vi "Create Image Name.vi"(8 "error in (no error)":errorcluster, 11 "Save Image in":refnum<class "Save Image.lvclass">) -> (0 "error out":errorcluster, 3 "Save Image out":refnum<class "Save Image.lvclass">)   [LabVIEW 2018, in "Save Image.lvclass"]
uses:
  Save Image.lvclass
  Save Image.lvclass/Save Image.ctl
  Simulated_Header/Simulated_Header.lvclass
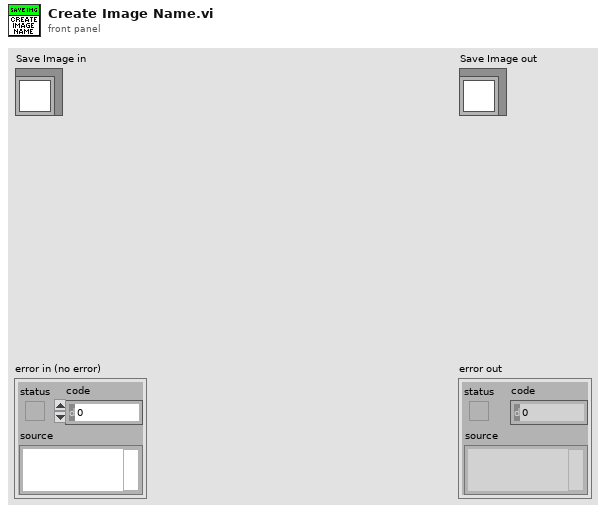
[diagram p1: front panel]
types:
  T1 = cluster{"COMNENT":string, "OBSTYPE":string, "ACSVRSN":string, "CHANNEL":u16, "LAST_IMG_NAME":string, "NIGHTDIR":string}
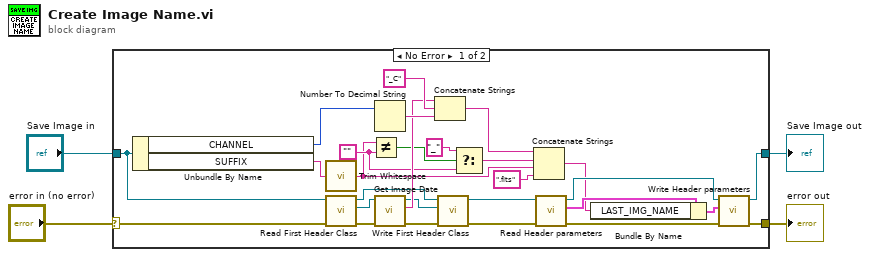
[diagram p0: block diagram]
diagram:
  n1 = case shown="No Error" "error in (no error)" {
    selector: "error in (no error)" -> [w16 w34]
    tunnel: [w12 w34] -> w3
    tunnel: [w13 w33] -> w1
    tunnel: "Save Image in" -> [w17 w33]
    frame No Error {
      w25 = ""
      n2 = Unbundle By Name(w17) -> ("CHANNEL"=w18:u16, "SUFFIX"=w23:string)
      n3 = call <vilib>:"Trim Whitespace.vi"("string"=w23) -> ("trimmed string"=w22:string)  [unwired: 1 in]
      n4 = call "Read First Header Class.vi"("error in (no error)"=w16, "Save Image in"=w17) -> ("error out"=w21:errorcluster, "Simulated_Header.lvclass"=w20:refnum<class "Simulated_Header.lvclass">, "Save Image out"=w19:refnum<class "Save Image.lvclass">)  [unwired: 7 in]
      n5 = Not Equal?(x=w22, y=w25) -> (x != y?=w28:bool)
      n6 = Number To Decimal String(number=w18) -> (decimal integer string=w31:string)  [unwired: 1 in]
      n7 = call-dynamic "Get Image Date.vi"("error in (no error)"=w21, "Simulated_Header in"=w20) -> ("error out"=w14:errorcluster, "Base image name"=w30:string, "Simulated_Header out"=w15:refnum<class "Simulated_Header.lvclass">)  [unwired: 7 in]
      n8 = Concatenate Strings(w30, "_C" ("string"), w31) -> (w29:string)
      n9 = call "Write First Header Class.vi"("error in (no error)"=w14, "Simulated_Header.lvclass"=w15, "Save Image in"=w19) -> ("error out"=w8:errorcluster, "Save Image out"=w9:refnum<class "Save Image.lvclass">)  [unwired: 7 in]
      n10 = Select(t="_" ("string"), s=w28, f=w25) -> (s? t:f=w26:string)
      n11 = Concatenate Strings(w29, w26, w22, ".fits" ("string")) -> (w5:string)
      n12 = call "Read Header parameters.vi"("error in (no error)"=w8, "Save Image in"=w9) -> ("error out"=w11:errorcluster, "Header parameters"=w6:T1, "Save Image out"=w10:refnum<class "Save Image.lvclass">)  [unwired: 7 in]
      n13 = Bundle By Name(cluster=w6, "LAST_IMG_NAME"=w5) -> (w7:T1)
      n14 = call "Write Header parameters.vi"("error in (no error)"=w11, "Header parameters"=w7, "Save Image in"=w10) -> ("error out"=w12:errorcluster, "Save Image out"=w13:refnum<class "Save Image.lvclass">)  [unwired: 7 in]
    }
    frame Error {
    }
  }
  "error out" <- w3
  "Save Image out" <- w1
